vi "参数设置对话框.vi"() -> ()   [LabVIEW 2016, in "德润DR803F超标留样.lvlib"]
uses:
  <vilib>/Utility/config.llb/NI_LVConfig.lvlib
panel:
  in  "读取":bool
  in  "设置":bool
  in  "VISA resource name":refnum<visa-resource-name>="COM10" caption="VISA资源名称"
  in  "关闭":bool
  in  "打开串口":bool
  in  "释放串口":bool
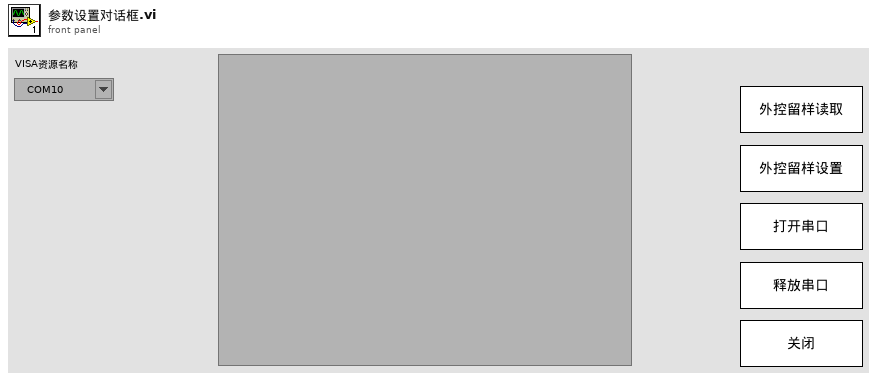
[diagram p1: front panel]
types:
  T1 = cluster{"枚举":enum16{"open", "read", "write", "close"}, "写入内容":string}
  T2 = enum32{"Bad", "Idle", "Run top level", "Running"}
  T3 = typedef "NI_LVConfig.lvlib/Config Data RefNum.ctl" = refnum<k1>
  T4 = cluster{"当前瓶号：":dbl, "平行样：":dbl, "留样瓶数：":dbl, "每瓶次数：":dbl, "每次留样：":dbl}
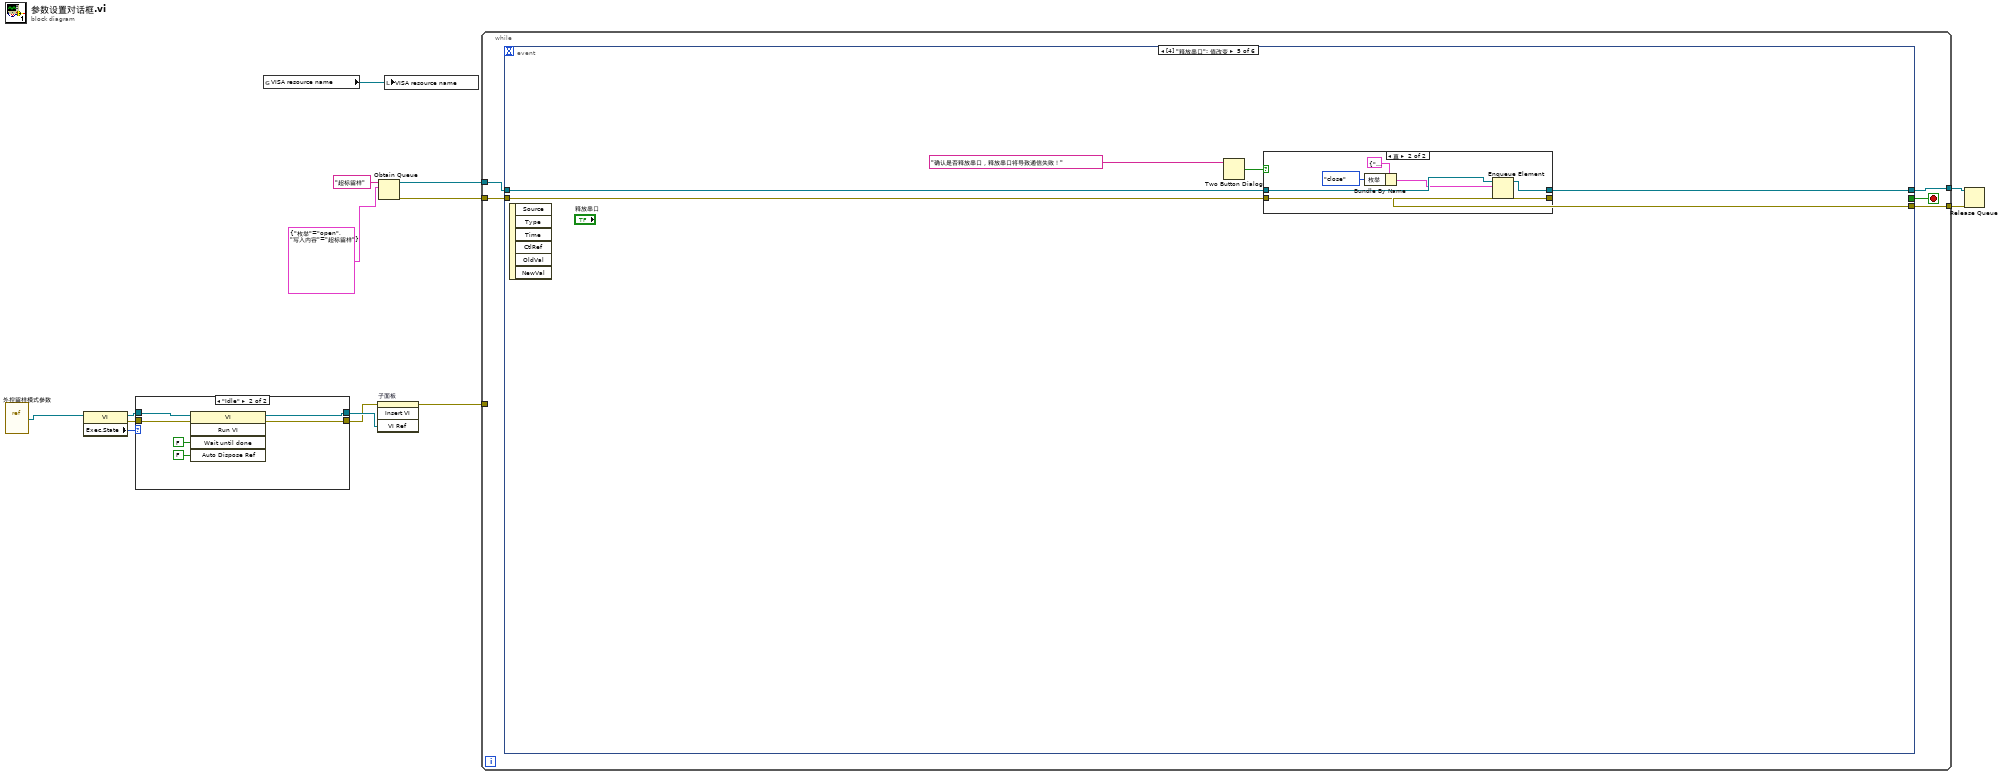
[diagram p0: block diagram]
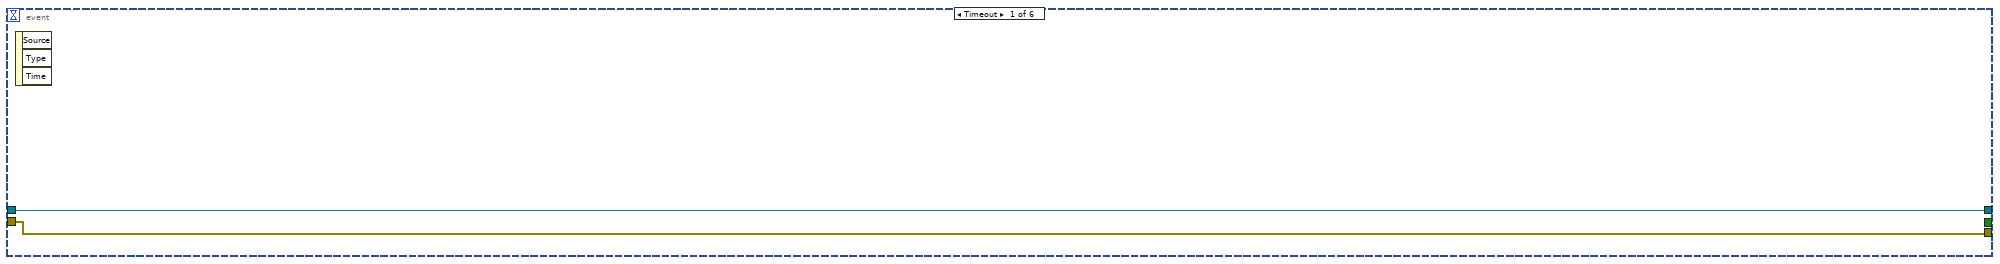
[diagram p3: hidden frame]
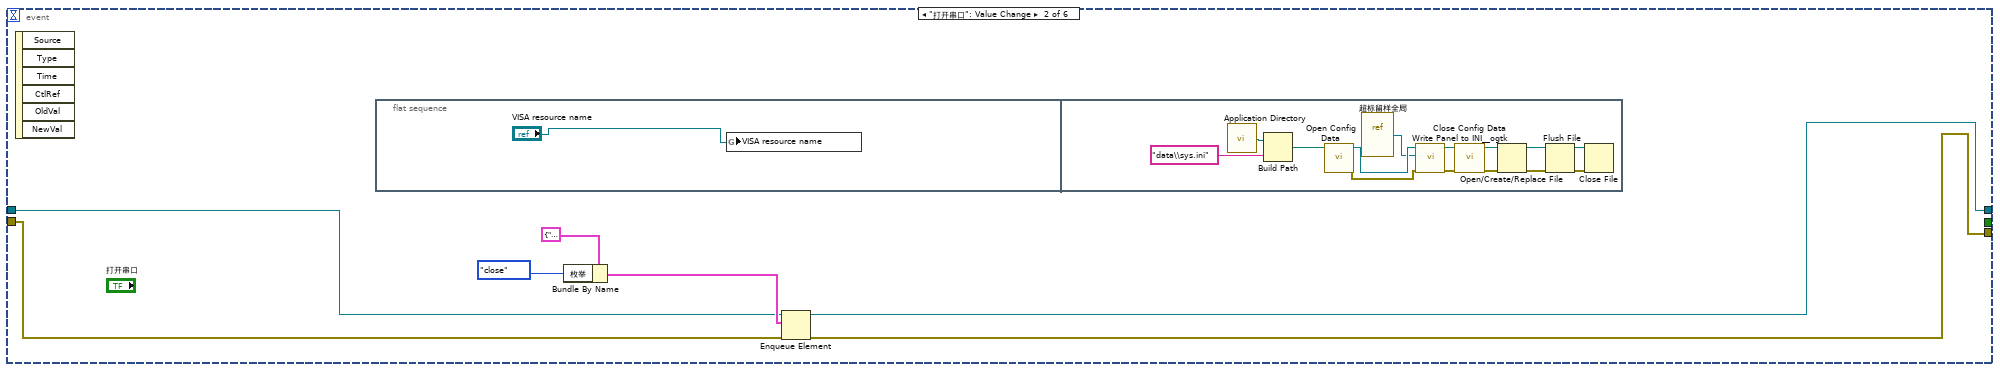
[diagram p4: hidden frame]
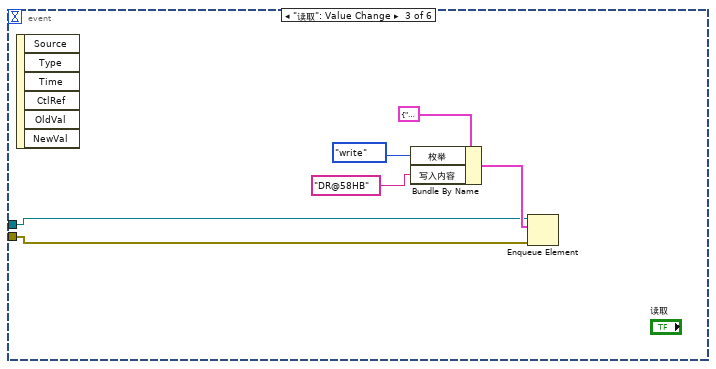
[diagram p5: hidden frame]
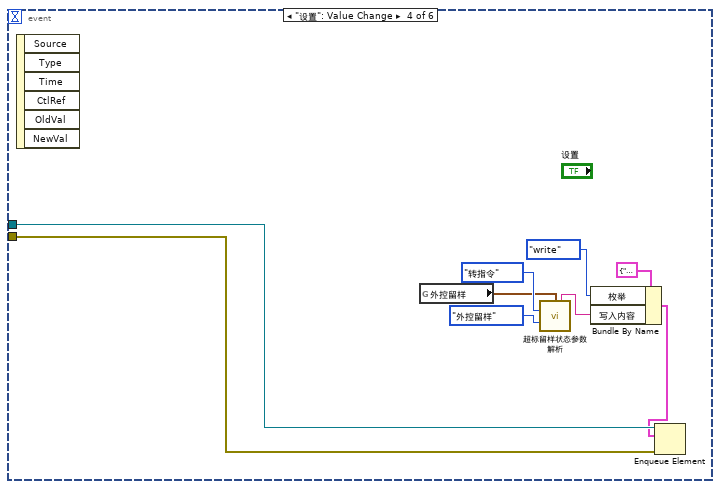
[diagram p6: hidden frame]
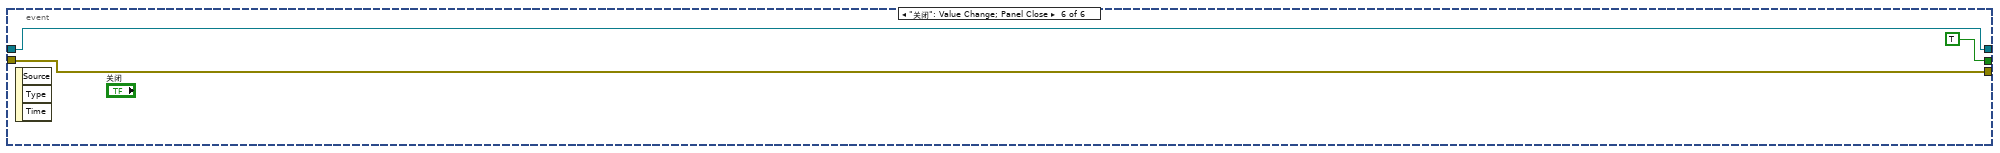
[diagram p8: hidden frame]
diagram:
  n1 = vi-ref "外控留样模式参数.vi"() -> (w1:refnum<vi>)
  n2 = property class="VI"(reference=w1) -> (reference out=w7:refnum<vi>, error out=w6:errorcluster, "Exec.State"=w8:T2)  [unwired: 1 in]
  n3 = case shown="\"Idle\"" w8 {
    tunnel: w7 -> [w16 w22]
    tunnel: [w16 w19] -> w5
    tunnel: w6 -> [w15 w18]
    tunnel: [w15 w17] -> w4
    frame "Bad", Default {
    }
    frame "Idle" {
      n4 = invoke class="VI" method="Run VI"(reference=w22, error in=w18, "Wait until done"=FALSE ("结束前等待"), "Auto Dispose Ref"=FALSE ("自动销毁引用")) -> (reference out=w19:refnum<vi>, error out=w17:errorcluster)  [unwired: 1 in, 3 out]
    }
  }
  n5 = global read "超标留样全局.vi" "VISA resource name"() -> (w2:refnum<visa-resource-name>)
  n6 = invoke on="子面板" class="SubPnl" method="Insert VI"(error in=w4, "VI Ref"=w5) -> (error out=w3:errorcluster)  [unwired: 2 in, 3 out]
  n7 = Obtain Queue(name (unnamed)="超标留样" ("名称（未命名）"), element data type=T1 {"枚举"=enum."open", "写入内容"="超标留样"}) -> (queue out=w10:refnum<queue>, error out=w9:errorcluster)  [unwired: 3 in, 1 out]
  n8 = local write "VISA resource name"(w2) -> ()
  n9 = while {
    tunnel: w10 -> [w27]
    tunnel: w9 -> [w26]
    tunnel: [w25] -> w13
    tunnel: [w24] -> w12
    tunnel: w3 -> [_]
    stop <- w23 stop-if-true
    n10 = event shown="[4] \"释放串口\": 值改变" {
      selector: _ -> [_ _ _ _ _ _]
      dyn-events: _ -> [_ _ _ _ _ _]
      timeout: _ -> [_ _ _ _ _ _]
      tunnel: w27 -> [w29 w33 w53 w66 w70 w83]
      tunnel: w26 -> [w28 w32 w52 w65 w69 w82]
      tunnel: [w29 w31 _ _ w68 w83] -> w25
      tunnel: [w28 w30 _ _ w67 w82] -> w24
      tunnel: [_ _ _ _ _ TRUE] -> w23
      event Timeout {
        n11 = event-data() -> ()  [unwired: 1 in, 3 out]
      }
      event "打开串口": Value Change {
        n12 = event-data() -> ()  [unwired: 1 in, 6 out]
        n13 = flat-sequence {
          frame #0 {
            n14 = global write "超标留样全局.vi" "VISA resource name"("VISA resource name") -> ()
          }
          frame #1 {
            n15 = call <vilib>:"Application Directory.vi"() -> ("Application Directory"=w40:path)
            n16 = Build Path(base path=w40, name or relative path="data\\sys.ini" ("名称或相对路径")) -> (appended path=w41:path)
            n17 = call <vilib>:"Open Config Data.vi"("configuration file path"=w41) -> ("error out"=w44:errorcluster, "refnum"=w42:T3)  [unwired: 8 in, 1 out]
            n18 = vi-ref "超标留样全局.vi"() -> (w38:refnum<vi>)
            n19 = call <userlib>:"Write Panel to INI__ogtk.vi"("error in (no error)"=w44, "VI ref"=w38, "refnum"=w42) -> ("error out"=w45:errorcluster, "refnum out"=w43:T3)  [unwired: 7 in]
            n20 = call <vilib>:"Close Config Data.vi"("error in (no error)"=w45, "refnum"=w43) -> ("error out"=w50:errorcluster, "file path"=w51:path)  [unwired: 8 in]
            n21 = Open/Create/Replace File(file path (use dialog)=w51, error in=w50) -> (refnum out=w47:refnum<file>, error out=w46:errorcluster)  [unwired: 4 in, 1 out]
            n22 = Flush File(refnum=w47, error in=w46) -> (refnum out=w48:refnum<file>, error out=w49:errorcluster)
            n23 = Close File(refnum=w48, error in=w49) -> ()  [unwired: 2 out]
          }
        }
        n24 = Bundle By Name(cluster=T1 {"枚举"=enum."open", "写入内容"="超标留样"}, "枚举"=enum16{"open", "read", "write", "close"}."close" ("元素")) -> (w34:T1)
        n25 = Enqueue Element(queue=w33, element=w34, error in (no error)=w32) -> (queue out=w31:refnum<queue>, error out=w30:errorcluster)  [unwired: 1 in, 1 out]
      }
      event "读取": Value Change {
        n26 = event-data() -> ()  [unwired: 1 in, 6 out]
        n27 = Bundle By Name(cluster=T1 {"枚举"=enum."open", "写入内容"="超标留样"}, "枚举"=enum16{"open", "read", "write", "close"}."write" ("元素"), "写入内容"="DR@58HB") -> (w57:T1)
        n28 = Enqueue Element(queue=w53, element=w57, error in (no error)=w52) -> ()  [unwired: 1 in, 3 out]
      }
      event "设置": Value Change {
        n29 = event-data() -> ()  [unwired: 1 in, 6 out]
        n30 = global read "超标留样全局.vi" "外控留样"() -> (w62:T4)
        n31 = call "超标留样状态参数解析.vi"("外控留样"=w62, "解析/转指令"=enum16{"解析", "转指令"}."转指令", "模式选择"=enum16{"外控留样", "超标留样"}."外控留样") -> ("输出字符串"=w59:string)  [unwired: 11 in, 1 out]
        n32 = Bundle By Name(cluster=T1 {"枚举"=enum."open", "写入内容"="超标留样"}, "枚举"=enum16{"open", "read", "write", "close"}."write" ("元素"), "写入内容"=w59) -> (w58:T1)
        n33 = Enqueue Element(queue=w66, element=w58, error in (no error)=w65) -> ()  [unwired: 1 in, 3 out]
      }
      event "释放串口": Value Change {
        n34 = event-data() -> ()  [unwired: 1 in, 6 out]
        n35 = Two Button Dialog(message="确认是否释放串口，释放串口将导致通信失败！" ("消息")) -> (T button?=w71:bool)  [unwired: 2 in]
        n36 = case shown="真" w71 {
          tunnel: w70 -> [w74 w81]
          tunnel: w69 -> [w73 w80]
          tunnel: [w74 w79] -> w68
          tunnel: [w73 w78] -> w67
          frame False {
          }
          frame True {
            n37 = Bundle By Name(cluster=T1 {"枚举"=enum."open", "写入内容"="超标留样"}, "枚举"=enum16{"open", "read", "write", "close"}."close" ("元素")) -> (w75:T1)
            n38 = Enqueue Element(queue=w81, element=w75, error in (no error)=w80) -> (queue out=w79:refnum<queue>, error out=w78:errorcluster)  [unwired: 1 in, 1 out]
          }
        }
      }
      event "关闭": Value Change; Panel Close {
        n39 = event-data() -> ()  [unwired: 1 in, 3 out]
      }
    }
  }
  n40 = Release Queue(queue=w13, error in (no error)=w12) -> ()  [unwired: 1 in, 3 out]
